vi "Engine-Event-WindowCloseRequested.vi"(8 "error in (no error)":errorcluster, 10 "Timestamp":u64, 11 "GLF Window in":refnum<class "Window.lvclass">) -> (0 "error out":errorcluster, 2 "Closed?":bool, 3 "GLF Window out":refnum<class "Window.lvclass">)   [LabVIEW 2020, in "GLF.lvlib" / "Window.lvclass"]
uses:
  Window.lvclass
  Window.lvclass/Window.ctl
  WindowEventInterface/WindowEventInterface.lvclass
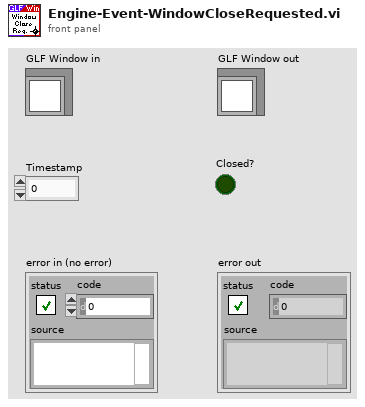
[diagram p1: front panel]
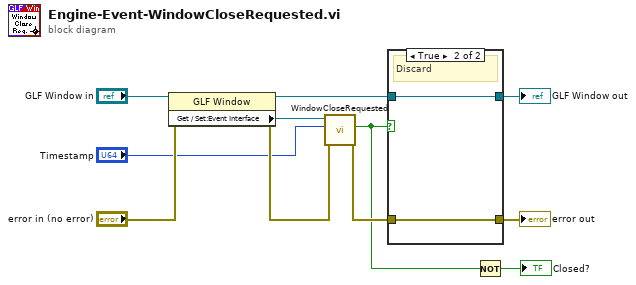
[diagram p0: block diagram]
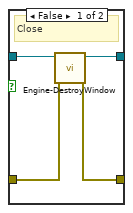
[diagram p2: hidden frame]
diagram:
  n1 = property class="GLF Window"(reference="GLF Window in", error in="error in (no error)") -> (reference out=w6:refnum<class "Window.lvclass">, error out=w8:errorcluster, "Get / Set:Event Interface"=w9:refnum<class "WindowEventInterface.lvclass">)
  n2 = call-dynamic "WindowCloseRequested.vi"("error in (no error)"=w8, "Timestamp"="Timestamp", "WindowEventInterface in"=w9) -> ("error out"=w4:errorcluster, "Discard?"=w2:bool)  [unwired: 7 in]
  n3 = case shown="True" w2 {
    tunnel: w6 -> [w15 w17]
    tunnel: [w14 w17] -> w5
    tunnel: w4 -> [w13 w16]
    tunnel: [w12 w16] -> w3
    frame False {
      # "Close"
      n4 = call "Engine-DestroyWindow.vi"("error in (no error)"=w13, "Window in"=w15) -> ("error out"=w12:errorcluster, "Window out"=w14:refnum<class "Window.lvclass">)  [unwired: 8 in]
    }
    frame True {
      # "Discard"
    }
  }
  "error out" <- w3
  "GLF Window out" <- w5
  n5 = Not(x=w2) -> (.not. x?=→"Closed?":bool)
